vi "DequeueMessage.vi"(8 "error in (no error)":errorcluster, 11 "DisplayBase in":refnum<class "DisplayBase.lvclass">) -> (0 "error out":errorcluster, 3 "String":string)   [LabVIEW 2020, in "DisplayBase.lvclass"]
uses:
  DisplayBase.lvclass
  DisplayBase.lvclass/DisplayBase.ctl
panel:
  # "Connector Pane"
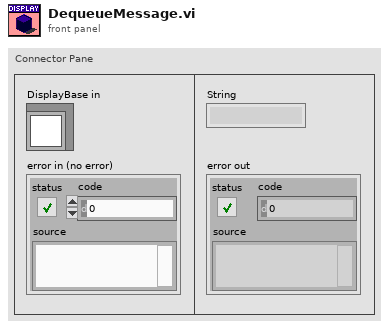
[diagram p1: front panel]
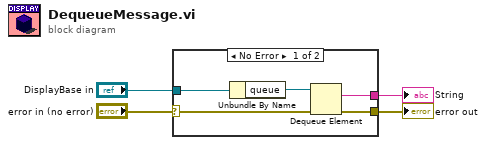
[diagram p0: block diagram]
diagram:
  n1 = case shown="No Error" "error in (no error)" {
    selector: "error in (no error)" -> [w5 w10]
    tunnel: "DisplayBase in" -> [w8 _]
    tunnel: [w7 w10] -> w3
    tunnel: [w6 _] -> w2
    frame No Error {
      n2 = Unbundle By Name(w8) -> ("queue"=w9:refnum<queue>)
      n3 = Dequeue Element(queue=w9, error in (no error)=w5) -> (element=w6:string, error out=w7:errorcluster)  [unwired: 1 in, 2 out]
    }
    frame Error {
    }
  }
  "error out" <- w3
  "String" <- w2
